vi "Remove Symbol Handle.vi"(8 "error in (no error)":errorcluster, 10 "Handle":i32, 11 "TwinCAT ADS in":refnum<class "TwinCAT ADS.lvclass">) -> (0 "error out":errorcluster, 3 "TwinCAT ADS out":refnum<class "TwinCAT ADS.lvclass">)   [LabVIEW 2018, in "TwinCAT ADS.lvclass"]
uses:
  TwinCAT ADS.lvclass
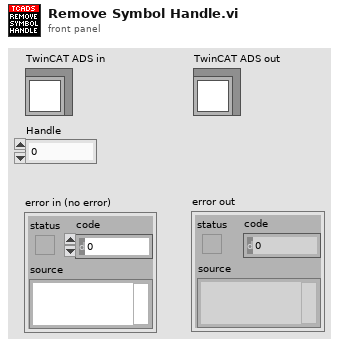
[diagram p1: front panel]
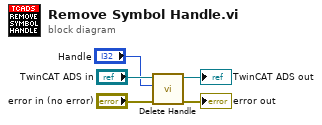
[diagram p0: block diagram]
diagram:
  n1 = call "Delete Handle.vi"("error in (no error)"="error in (no error)", "Handle"="Handle", "TwinCAT ADS in"="TwinCAT ADS in") -> ("error out"=→"error out":errorcluster, "TwinCAT ADS out"=→"TwinCAT ADS out":refnum<class "TwinCAT ADS.lvclass">)  [unwired: 7 in]
